vi "UMLEditor_GetActiveWindowDLL.vi"() -> (2 "Active Window":string)   [LabVIEW 2020]
uses:
  user32.dll
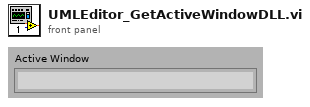
[diagram p1: front panel]
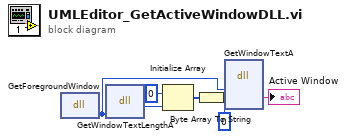
[diagram p0: block diagram]
diagram:
  n1 = dll-call lib="user32.dll" fn="GetForegroundWindow"() -> (w2:u32)  [unwired: 3 in, 2 out]
  n2 = dll-call lib="user32.dll" fn="GetWindowTextLengthA"("whnd"=w2) -> (w4:i32)  [unwired: 4 in, 2 out]
  n3 = Initialize Array(u8 0, w4) -> (w6:u8[])
  n4 = Byte Array To String(unsigned byte array=w6) -> (string=w5:string)
  n5 = dll-call lib="user32.dll" fn="GetWindowTextA"("HWND"=w2, "Title"=w5, "StringLength"=0) -> ("Title"=→"Active Window":string)  [unwired: 4 in, 4 out]
